vi "Update Timing Statistics.vi"(8 "error in (no error)":errorcluster, 9 "Time to Add":dbl, 10 "Qualified Name":string, 11 "ResultTree in":refnum<class "ResultTree.lvclass">) -> (0 "error out":errorcluster, 1 "Total Time":dbl, 3 "ResultTree out":refnum<class "ResultTree.lvclass">)   [LabVIEW 2017, in "ResultTree.lvclass"]
uses:
  ResultTree.lvclass
  ResultTree.lvclass/ResultTree.ctl
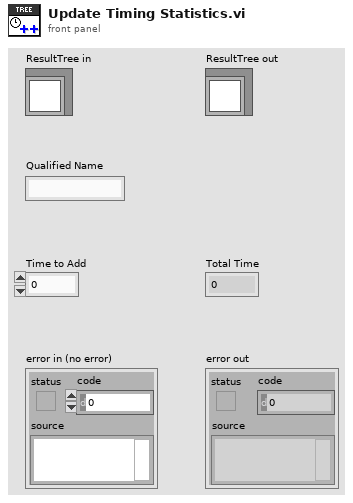
[diagram p1: front panel]
types:
  T1 = cluster{"Qualified Name":string, "Duration":dbl}[]
  T2 = cluster{"Qualified Name":string, "Time to Add":dbl}
  T3 = cluster{"Qualified Name":string, "Time to Add":dbl}[]
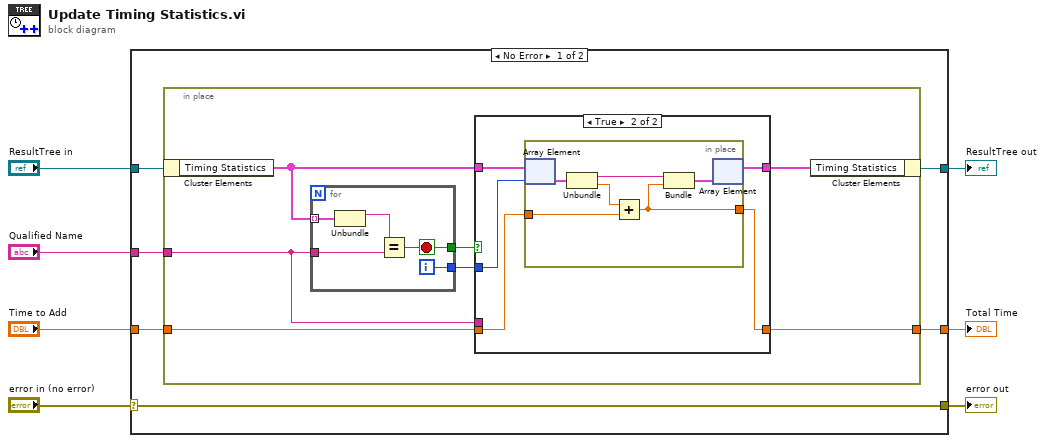
[diagram p0: block diagram]
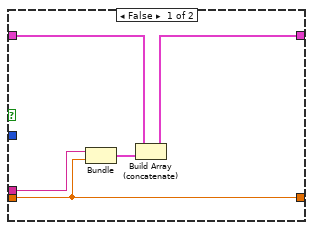
[diagram p2: hidden frame]
diagram:
  n1 = case shown="No Error" "error in (no error)" {
    selector: "error in (no error)" -> [w13 w43]
    tunnel: [w13 w43] -> w6
    tunnel: [w9 w42] -> w4
    tunnel: "ResultTree in" -> [w12 w42]
    tunnel: "Qualified Name" -> [w11 _]
    tunnel: "Time to Add" -> [w10 _]
    tunnel: [w8 _] -> w1
    frame No Error {
      n2 = in-place {
        in-place-border: w11 -> [w15]
        in-place-border: w10 -> [w16]
        in-place-border: [w14] -> w8
        n3 = in-place-cluster #1(w12) -> ("Timing Statistics"=w17:T1)
        n4 = for {
          tunnel: w17 -> [w41] mode=indexing
          tunnel: w15 -> [w39]
          tunnel: [w38] -> w20
          tunnel: [w37] -> w19
          i -> [w37]
          stop <- w38 stop-if-true
          n5 = Unbundle(w41) -> ("Qualified Name"=w40:string)  [unwired: 1 out]
          n6 = Equal?(x=w40, y=w39) -> (x = y?=w38:bool)
        }
        n7 = case shown="True" w20 {
          tunnel: w19 -> [_ w28]
          tunnel: w17 -> [w25 w30]
          tunnel: w16 -> [w21 w29]
          tunnel: [w22 w27] -> w18
          tunnel: w15 -> [w24 _]
          tunnel: [w21 w26] -> w14
          frame False {
            n8 = Bundle("Qualified Name"=w24, "Time to Add"=w21) -> (w23:T2)  [unwired: 1 in]
            n9 = Build Array (concatenate)(w25, w23) -> (w22:T3)
          }
          frame True {
            n10 = in-place {
              in-place-border: w29 -> [w32]
              in-place-border: [w31] -> w26
              n11 = in-place-array #2(w30, w28) -> (w36:cluster{"Qualified Name":string, "Duration":dbl})
              n12 = Unbundle(w36) -> ("Qualified Name"=w35:string, "Duration"=w33:dbl)
              n13 = Add(x=w33, y=w32) -> (x+y=w31:dbl)
              n14 = Bundle("Qualified Name"=w35, w31) -> (w34:cluster{"Qualified Name":string, dbl})  [unwired: 1 in]
              n15 = in-place-array #2(w34) -> (w27:T1)  [unwired: 1 out]
            }
          }
        }
        n16 = in-place-cluster #1("Timing Statistics"=w18) -> (w9:refnum<class "ResultTree.lvclass">)
      }
    }
    frame Error {
    }
  }
  "error out" <- w6
  "ResultTree out" <- w4
  "Total Time" <- w1
